vi "Test Async.vi"(10 "ExecAnchor":refnum<class "ExecAnchor.lvclass">) -> ()   [LabVIEW 2020]
uses:
  ExecAnchor/ExecAnchor.lvclass
panel:
  out "Count":i32
  # "Close the main VI and this should close as well."
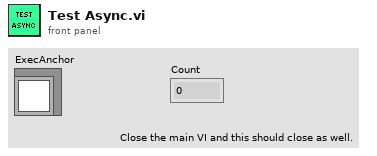
[diagram p1: front panel]
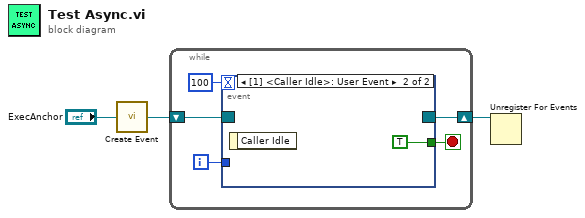
[diagram p0: block diagram]
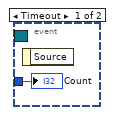
[diagram p2: hidden frame]
diagram:
  n1 = call "Create Event.vi"("ExecAnchor in"="ExecAnchor") -> ("Event Reg"=w2:refnum<event-registration>)  [unwired: 3 in, 1 out]
  n2 = while {
    shift-right: [w5] -> w1
    shift-left: w2 -> [w6]
    i -> [w7]
    stop <- w4 stop-if-true
    n3 = event shown="[1] <Caller Idle>: User Event" {
      selector: w6 -> [_ _]
      dyn-events: [_ _] -> w5
      timeout: 100 -> [_ _]
      tunnel: w7 -> [w9 _]
      tunnel: [_ TRUE] -> w4
      event Timeout {
        n4 = event-data() -> ()  [unwired: 1 in, 1 out]
        "Count" <- w9
      }
      event User Event {
        n5 = event-data() -> ()  [unwired: 1 in, 1 out]
      }
    }
  }
  n6 = Unregister For Events(event registration refnum=w1) -> ()  [unwired: 1 in, 1 out]
